vi "Handle Error.vi"(8 "error in (no error)":errorcluster, 11 "Sim Display Console Actor in":refnum<class "Sim Display Console Actor.lvclass">) -> (0 "error out":errorcluster, 2 "stop actor?":bool=TRUE, 3 "Sim Display Console Actor out":refnum<class "Sim Display Console Actor.lvclass">)   [LabVIEW 2022 SP3, in "Sim Display Console Actor.lvlib" / "Sim Display Console Actor.lvclass"]
doc: "(<B>Filename</B>: Actor Framework.lvlib:Actor.lvclass:Handle Error.vi)\n\nDefines how the actor handles an error that occurred while processing a message.\n\nBy default, this method does nothing except stop the actor. This method also treats error code 43 (coming from <B>error in</B>) as a sign that the actor shut down normally. In this situation, the Handle Error method does not return the error on <B>error out</B>, meaning the actor's caller will not receive it. All other error codes will be returned on <B>error out</B>.\n\nA descendant class may override this method to change this behavior."
uses:
  Sim Display Console Actor.lvclass
  Sim Display Console Actor.lvclass/Sim Display Console Actor.ctl
  Display Console Actor/Display Console Actor/Display Console Actor.lvclass
  <vilib>/ActorFramework/Actor/Actor.lvclass
  Interface Elevator/Interface Elevator Messages/Execute Error Handling Msg/Execute Error Handling Msg.lvclass
  Elevator Controller Actor/Elevator Controller Actor/Error Level.ctl
  Elevator Controller Actor/Elevator Controller Actor/Elevator Controller Actor.lvclass
  C:/Workspace/CLA/Elevator AF_2022_2nd/Display Console Actor/Display Console Actor/Display Console Actor.lvclass
  C:/Program Files/National Instruments/LabVIEW 2022/vi.lib/ActorFramework/Actor/Actor.lvclass
  C:/Workspace/CLA/Elevator AF_2022_2nd/Sim Display Console Actor/Elevator Controller Actor/Sim Display Console Actor.lvclass
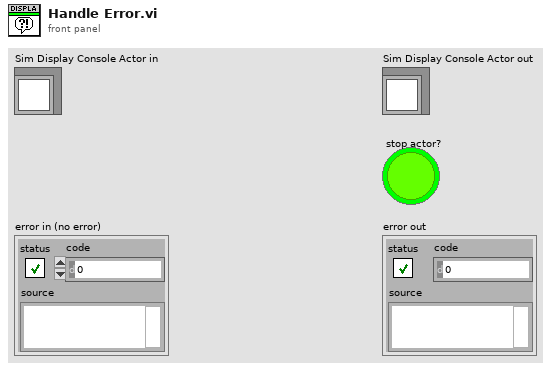
[diagram p1: front panel]
types:
  T1 = typedef "Elevator Controller Actor.lvlib/Elevator Controller Actor.lvclass/Error Level.ctl" = enum16{"Console Error", "Sensor Interface IO Error", "Process Step Error"}
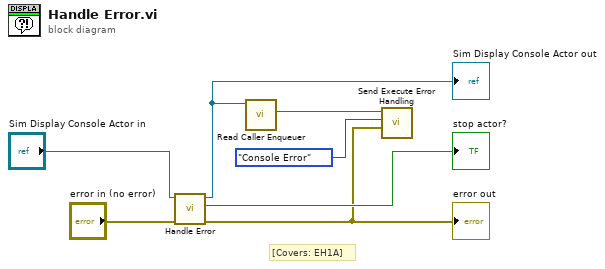
[diagram p0: block diagram]
diagram:
  # "[Covers: EH1A]"
  n1 = call-parent "Handle Error.vi"("error in (no error)"="error in (no error)", "Actor in"="Sim Display Console Actor in") -> ("error out"=w3:errorcluster, "stop actor?"=→"stop actor?":bool, "Actor out"=w1:refnum<class "Sim Display Console Actor.lvclass">)  [unwired: 7 in]
  "Sim Display Console Actor out" <- w1
  "error out" <- w3
  n2 = call <vilib>:"Read Caller Enqueuer.vi"("Actor"=w1) -> ("Caller Enqueuer"=w2:refnum<class "Message Enqueuer.lvclass">)  [unwired: 10 in]
  n3 = call "Send Execute Error Handling.vi"("Error"=w3, "Error Level"=Error_Level."Console Error", "Message Enqueuer"=w2) -> ()  [unwired: 7 in, 2 out]
